vi "Target Configuration.vi"() -> ()   [LabVIEW 2019, in "LMH-LINX.lvlib"]
uses:
  <vilib>/MakerHub/LINX/LMH-LINX.lvlib
  <vilib>/MakerHub/LINX/Private/Utilties/Target Management/Install LV Data.ctl
  <vilib>/MakerHub/LINX/Private/Utilties/Target Management/Target Info.ctl
  <vilib>/MakerHub/LINX/Private/Utilties/Target Management/NIC Info.ctl
  <vilib>/MakerHub/LINX/Private/Utilties/Target Management/NIC Mode.ctl
  <vilib>/MakerHub/LINX/Private/Utilties/Install LV Events.ctl
  <vilib>/MakerHub/LINX/Private/Utilties/Target Management/Status FGV States.ctl
  <vilib>/MakerHub/LINX/Private/Utilties/Target Management/Network Settings Ctrl Refs.ctl
  <vilib>/MakerHub/LINX/Private/Utilties/Target Management/Generic FGV State.ctl
  <vilib>/Platform/browser.llb/Open URL in Default Browser (path).vi
  <vilib>/Platform/browser.llb/Open URL in Default Browser (string).vi
  <vilib>/MakerHub/Toolbox/LMH-Toolbox.lvlib
panel:
  out "Target Status 2":string
  in  "View Log":bool
  out "Status Hostname":string
  out "Target Icon":u16(ring)
  in  "Target Info":bool
  in  "Cancel All":bool=TRUE
  in  "Network Settings":bool
  in  "Installation":bool
  in  "Connection":bool=TRUE
  in  "Main OK":bool
  out "Live Status":string="Successfully connected."
  out "Error Out":errorcluster
  in  "Tab Control":T1(tab)
  out "BBB Info":bool caption="Connect your device using both USB and ethernet.\n\nUsername and password need to have sudo privileges on the target - 'debian' and 'temppwd' are the default.\n\nThe mounted USB drive includes a START.htm guide."
  out "RPI Info":bool caption="Connect your device via ethernet.\n\nUse a monitor and mouse to enable SSH.\n\nUsername and password need to have sudo privileges on the target - 'pi' and 'raspberry' are the default."
  in  "Additional installation information:":bool
  in  "Hostname or IP:":string="raspberrypi"
  in  "Username:":string="pi"
  in  "Password:":string="raspberry"
  in  "Connect":bool
  in  "Target Type":u16(ring) items=["Raspberry Pi", "BeagleBone Black"]
  out "Update Available":string="Update Available"
  in  "Install":bool
  out "Installed Version:":string
  out "Available Version:":string="14.1-9"
  in  "Example":bool
  out "EULA Link":string="here"
  in  "Network Interface:":u16(ring) items=["", "lo:", "wlan0:"]
  in  "Default gateway:":string
  in  "Subnet mask:":string
  in  "IP address:":string
  in  "Password:":string
  in  "SSID:":string
  in  "Network Settings Save":bool
  in  "Network Settings Cancel":bool
  in  "DCHP":enum32{"DHCP", "Static"}(radio)
  in  "NIC Status":string
  in  "Hostname:":string="mypi\n"
  out "Target Status":string
  out "Internet Access":string="Internet Access Confirmed"
  out "CPU Info:":string
  out "OS Version:":string="8.0\n"
  # "Wifi Settings"
  # "General Settings"
  # "IP Addresses:"
  # "Note: This utility is designed for configuring idle network adapters only.   Using it to configure an active \n           network adapter is not recommended and may result in loss of connectivity."
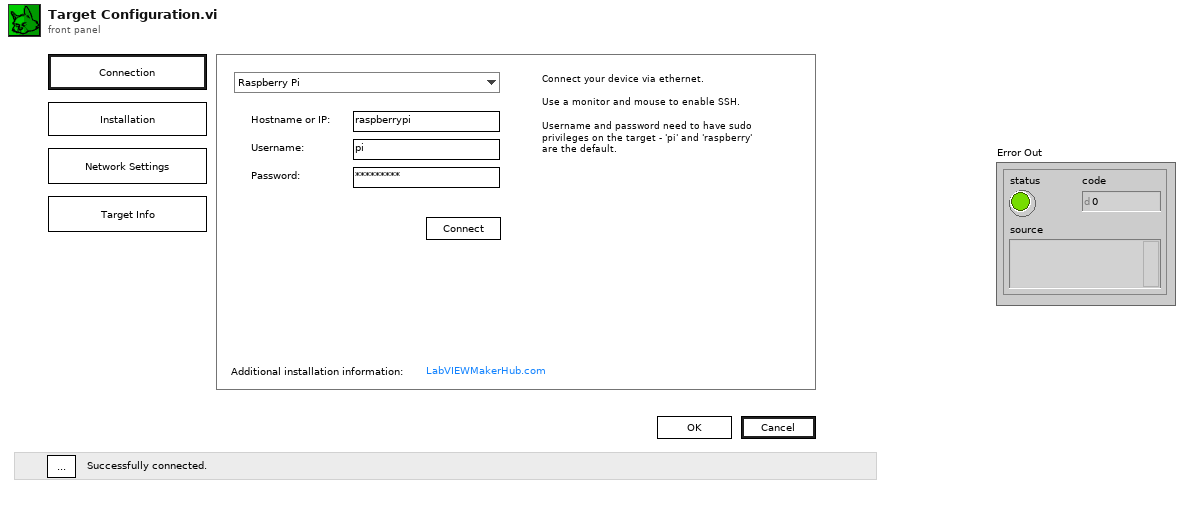
[diagram p1: front panel]
types:
  T1 = enum32{"Target", "Software", "Network", "Target Info"}
  T2 = typedef "LMH-LINX.lvlib/Install LV Events.ctl" = enum16{"Idle", "Connect", "Interrogate Device", "Pre Install", "Add MakerHub Feed", "Update Package Index", "Install LV", "Start LV", "Launch Example", "View Log", "Exit", "Update Hostname", "Menu: Target", "Menu: Install Software", "Menu: Network Settings", "Menu: Target Info", "NIC Select Change", "Menu: Network Settings Save", "Menu: Network Settings Cancel", "Menu: Cancel All"}
  T3 = typedef "LMH-LINX.lvlib/Install LV Data.ctl" = cluster{"SSH Session":refnum<k1>, "Status Log":string, "Detailed Log":string, "Credentials":cluster{"Hostname or IP":string, "Username":string, "Password":string}, "Target Info":T4, "Reboot Required?":bool}
  T4 = typedef "LMH-LINX.lvlib/Target Info.ctl" = cluster{"OS Version":string, "CPU":string, "Systemd Version":string, "Internet Access":bool, "Device Type":string, "LV Installed Ver":string, "LV Available Ver":string, "LV Upgrade Available":bool, "Hostname":string, "NIC Info":T5[]}
  T5 = typedef "LMH-LINX.lvlib/NIC Info.ctl" = cluster{"Name":string, "NIC Mode":T6, "Configured":bool, "Config IP address":string, "Config Subnet mask":string, "Config Network":string, "Config gateway":string, "Wifi":bool, "SSID":string, "Password":string, "Configuration":string, "Current IP address":string, "Current Subnet mask":string, "Current gateway":string, "Current Network":string}
  T6 = typedef "LMH-LINX.lvlib/NIC Mode.ctl" = enum16{"DHCP", "Static", "Loopback"}
  T7 = enum8{"Enabled", "Disabled", "Disabled and Grayed Out"}
  T8 = typedef "LMH-LINX.lvlib/Generic FGV State.ctl" = enum16{"Get", "Set"}
  T9 = typedef "LMH-LINX.lvlib/Network Settings Ctrl Refs.ctl" = cluster{"Hostname":refnum<vi>, "IP address":refnum<vi>, "Subnet mask":refnum<vi>, "Default Gateway":refnum<vi>, "SSID":refnum<vi>, "Password":refnum<vi>, "NIC Status":refnum<vi>, "Network Interface":refnum<vi>, "DCHP":refnum<vi>}
  T10 = typedef "LMH-LINX.lvlib/Status FGV States.ctl" = enum16{"Init", "Append", "Append History Only", "Set", "Get"}
  T11 = typedef "LMH-LINX.lvlib/Target Compatibility Warnings.ctl" = cluster{"Warning?":bool, "Details":string, "Help URL":string, "Fix It Button Name":string, "Fix It VI Ref":refnum<vi>}
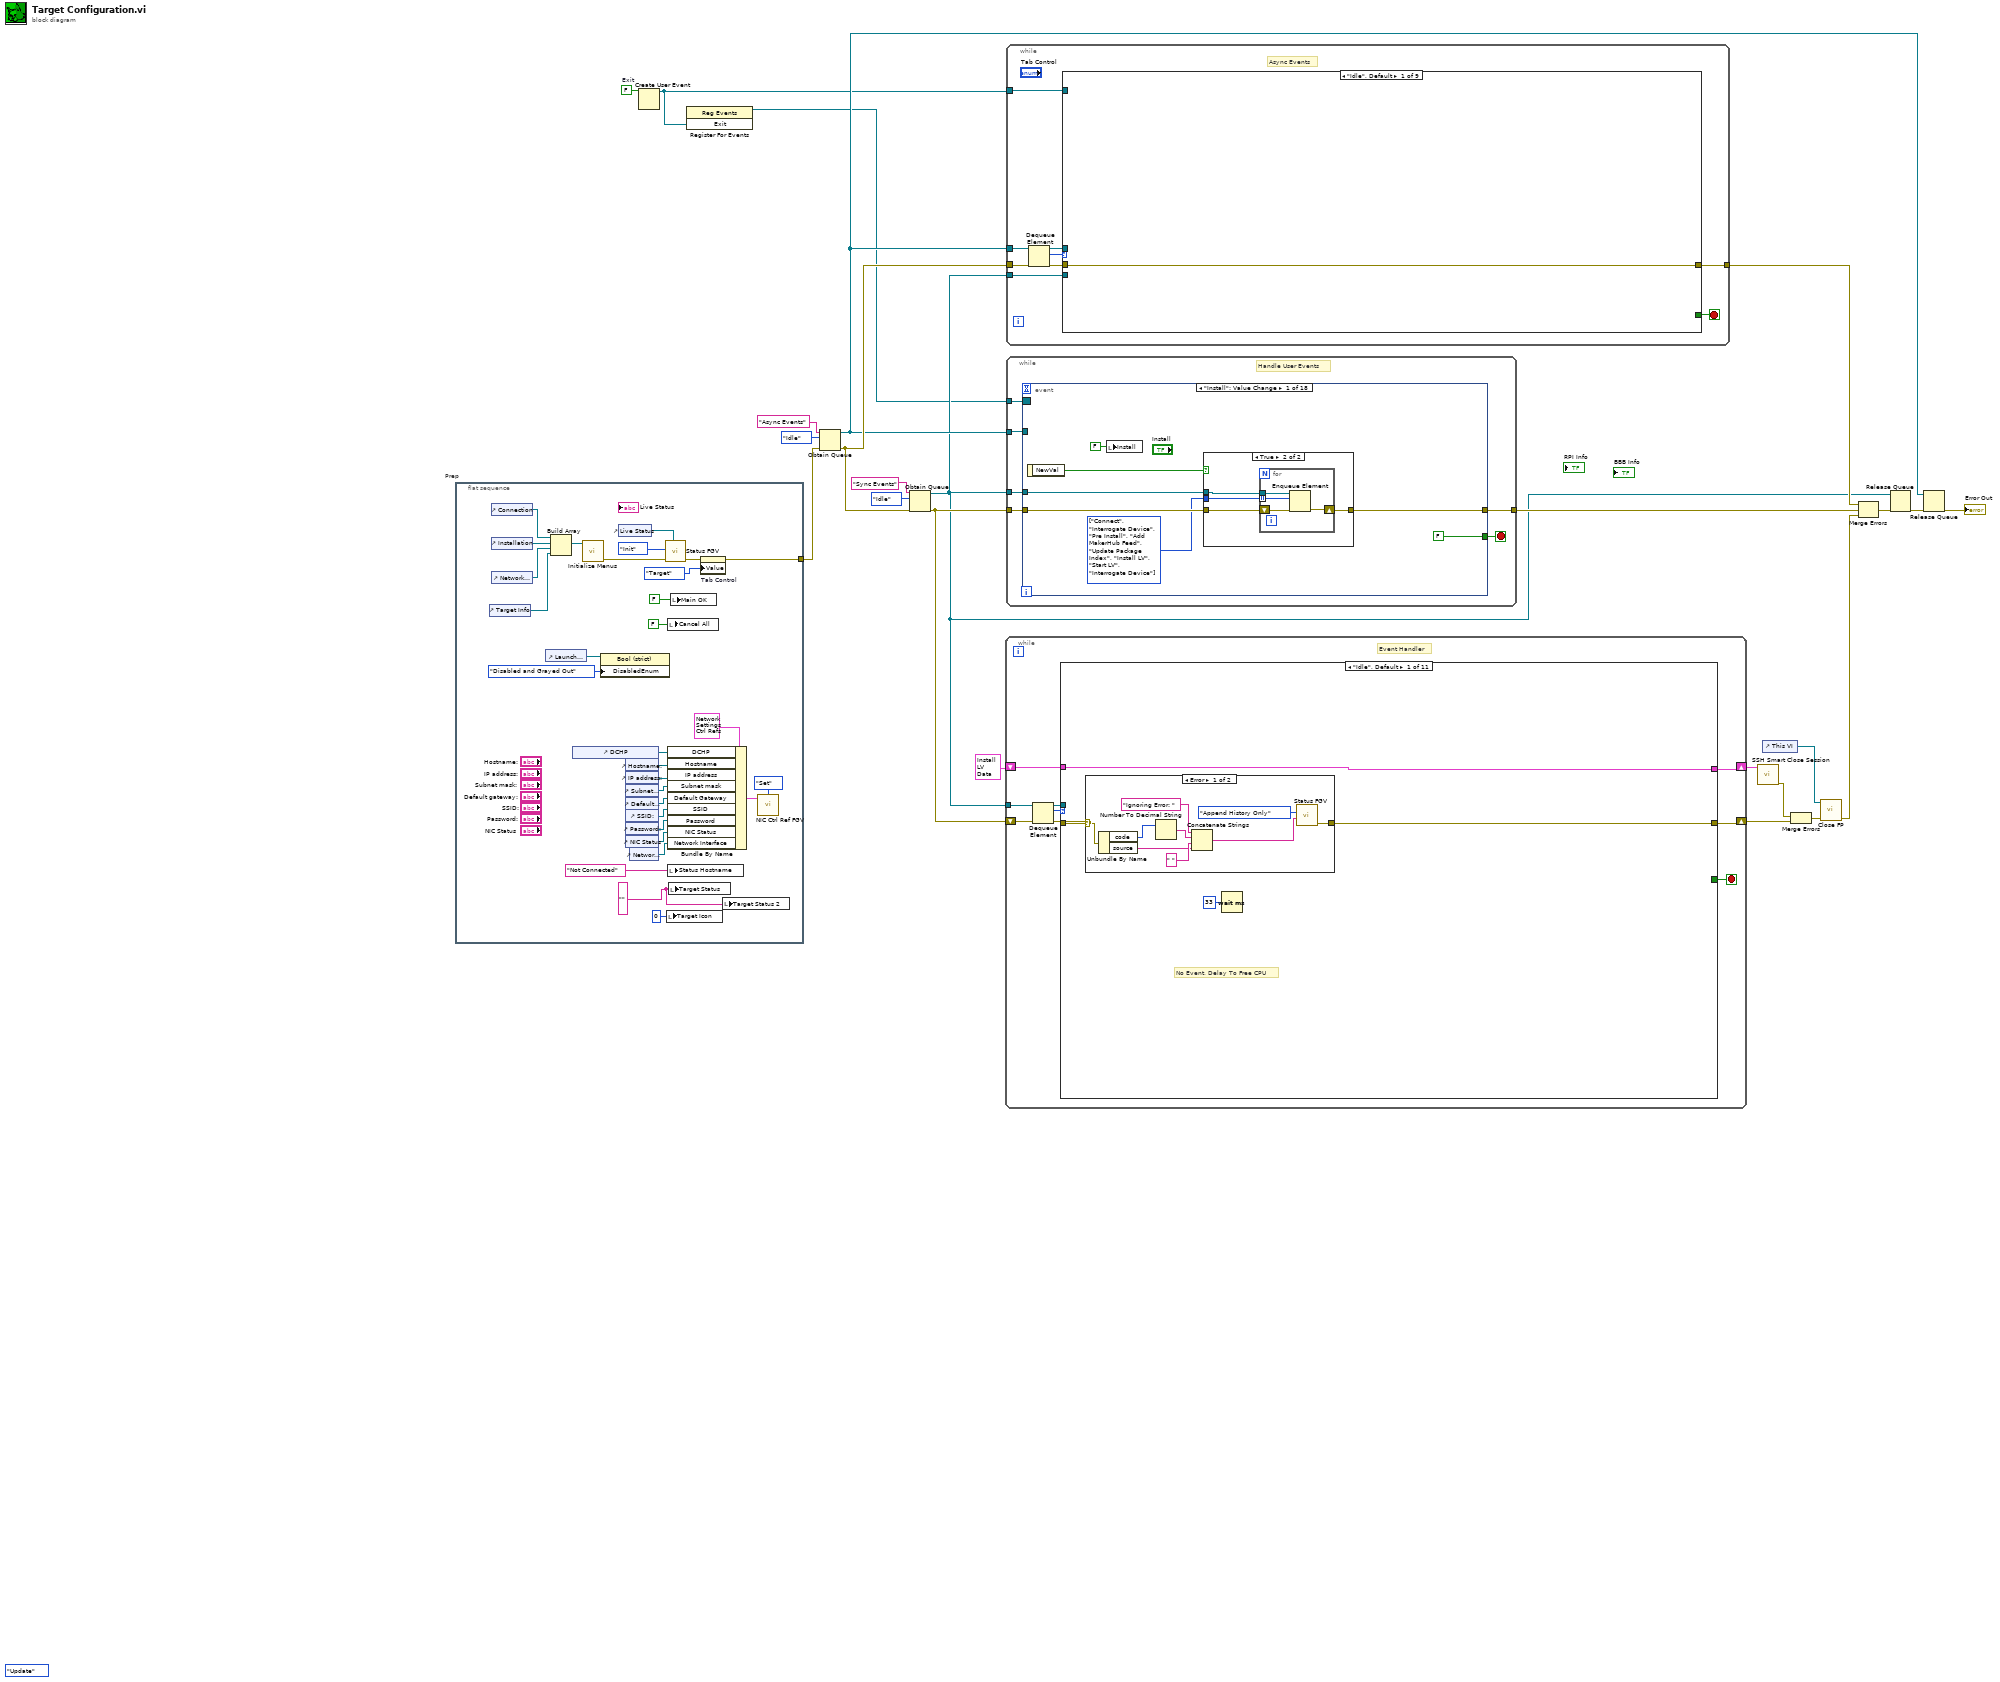
[diagram p0: block diagram]
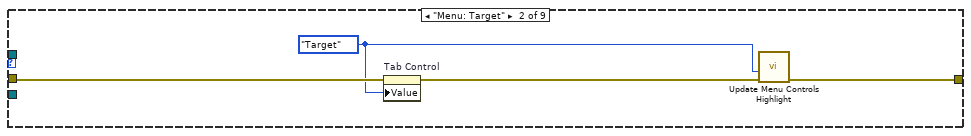
[diagram p2: hidden frame]
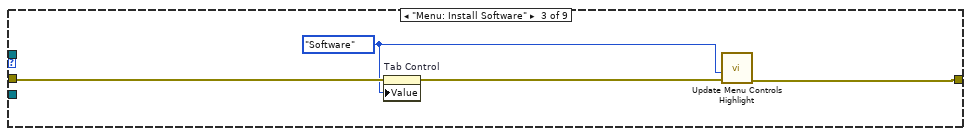
[diagram p3: hidden frame]
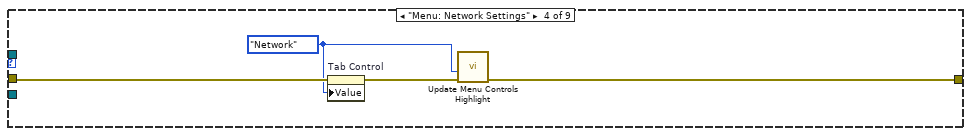
[diagram p4: hidden frame]
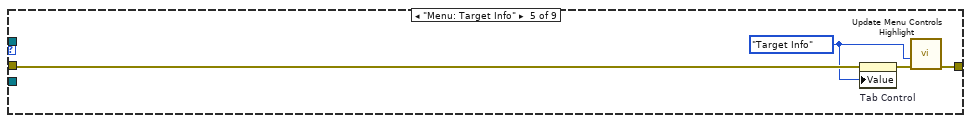
[diagram p5: hidden frame]
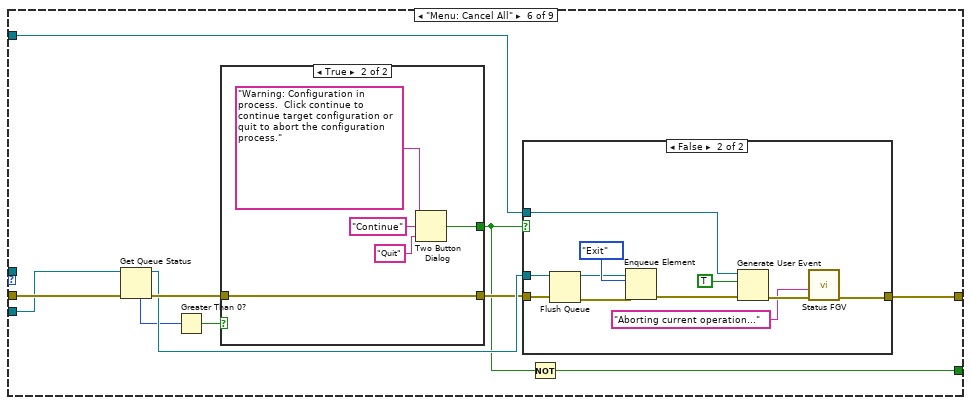
[diagram p6: hidden frame]
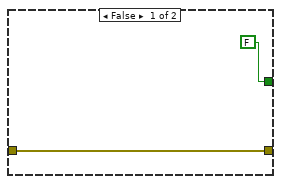
[diagram p8: hidden frame]
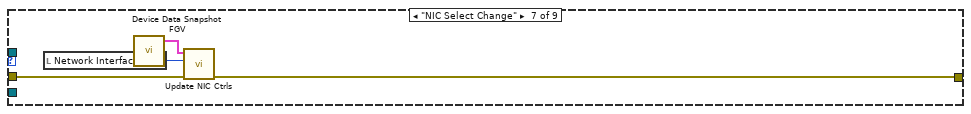
[diagram p9: hidden frame]
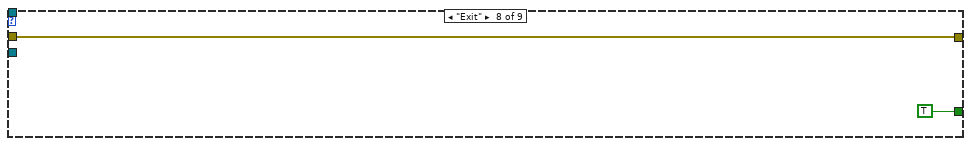
[diagram p10: hidden frame]
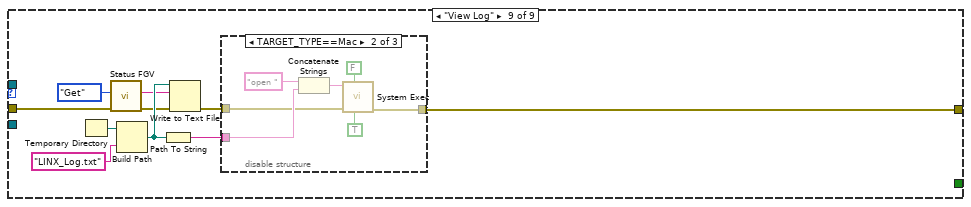
[diagram p11: hidden frame]
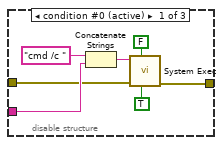
[diagram p12: hidden frame]
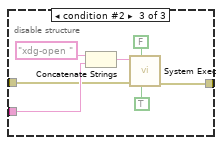
[diagram p13: hidden frame]
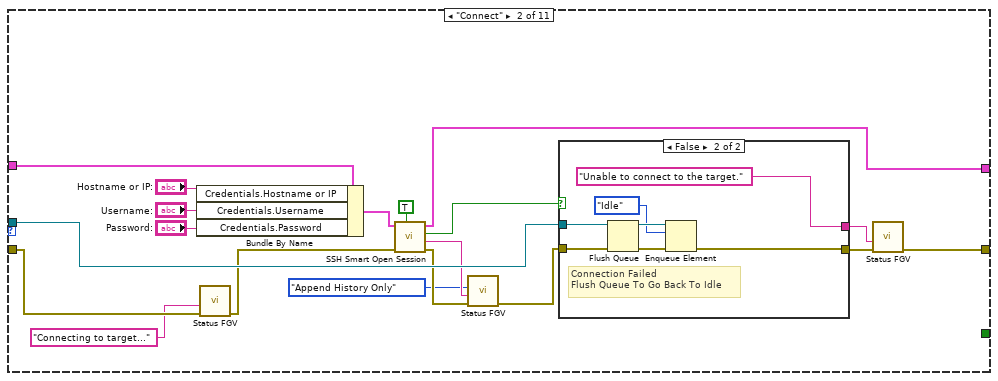
[diagram p15: hidden frame]
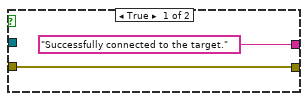
[diagram p16: hidden frame]
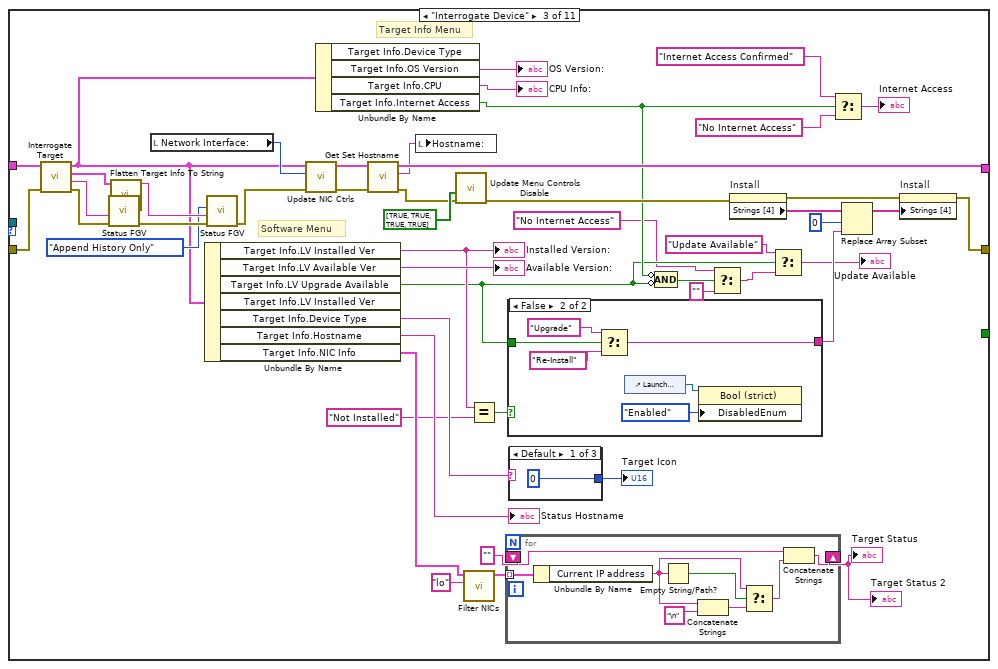
[diagram p17: hidden frame]
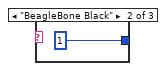
[diagram p18: hidden frame]
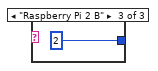
[diagram p19: hidden frame]
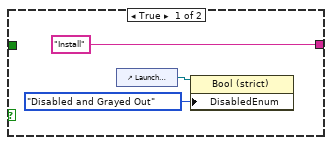
[diagram p20: hidden frame]
diagram:
  w8 = FALSE  # Exit
  (unwired) enum16{"Init", "Update"}."Update"
  n1 = flat-sequence "Prep" {
    tunnel: [w44] -> w2
    frame #0 {
      w25 = "" ("Target Stats")
      n2 = control-ref of="Target Info"() -> (w46:refnum<vi>)
      n3 = control-ref of="Connection"() -> (w51:refnum<vi>)
      n4 = control-ref of="Installation"() -> (w50:refnum<vi>)
      n5 = control-ref of="Network Settings"() -> (w49:refnum<vi>)
      n6 = control-ref of="Launch Example"() -> (w28:refnum<vi>)
      n7 = Build Array(w51, w50, w49, w46) -> (w48:refnum<vi>[])
      n8 = control-ref of="DCHP"() -> (w36:refnum<vi>)
      n9 = call <vilib>:"Initialize Menus.vi"("Menu Controls"=w48) -> ("Error Out"=w47:errorcluster)  [unwired: 10 in]
      n10 = property class="Bool (strict)"(reference=w28, "DisabledEnum"=T7."Disabled and Grayed Out" ("Disabled")) -> ()  [unwired: 1 in, 2 out]
      n11 = control-ref of="Live Status"() -> (w53:refnum<vi>)
      n12 = control-ref of="Hostname:"() -> (w31:refnum<vi>)
      n13 = control-ref of="IP address:"() -> (w37:refnum<vi>)
      n14 = control-ref of="Subnet mask:"() -> (w38:refnum<vi>)
      n15 = control-ref of="Default gateway:"() -> (w39:refnum<vi>)
      n16 = control-ref of="SSID:"() -> (w40:refnum<vi>)
      n17 = control-ref of="Password:"() -> (w41:refnum<vi>)
      n18 = control-ref of="NIC Status"() -> (w42:refnum<vi>)
      n19 = control-ref of="Network Interface:"() -> (w34:refnum<vi>)
      n20 = call <vilib>:"Status FGV.vi"("Live Status Ref"=w53, "Error In"=w47, "Status FGV State"=Status_FGV_States."Init") -> ("Error Out"=w45:errorcluster)  [unwired: 6 in, 2 out]
      n21 = local write "Target Icon"(u16 0 ("Target Icon")) -> ()
      n22 = local write "Cancel All"(FALSE ("Stop Button")) -> ()
      n23 = Bundle By Name(cluster=T9 {"Hostname"=refnum, "IP address"=refnum, "Subnet mask"=refnum, "Default Gateway"=refnum, "SSID"=refnum, "Password"=refnum, "NIC Status"=refnum, "Network Interface"=refnum, "DCHP"=refnum} ("Network Settings Ctrl Refs"), "DCHP"=w36, "Hostname"=w31, "IP address"=w37, "Subnet mask"=w38, "Default Gateway"=w39, "SSID"=w40, "Password"=w41, "NIC Status"=w42, "Network Interface"=w34) -> (w33:T9)
      n24 = local write "Status Hostname"("Not Connected") -> ()
      n25 = local write "Target Status"(w25) -> ()
      n26 = local write "Main OK"(FALSE ("Stop Button")) -> ()
      n27 = property on="Tab Control" class="TabCtl (strict)"(error in=w45, "Value"=T1."Target" ("Tab Control")) -> (error out=w44:errorcluster)  [unwired: 1 in, 1 out]
      n28 = local write "Target Status 2"(w25) -> ()
      n29 = call <vilib>:"NIC Ctrl Ref FGV.vi"("Network Settings Ctrl Refs"=w33, "FGV State"=Generic_FGV_State."Set") -> ()  [unwired: 2 in, 1 out]
    }
  }
  n30 = Create User Event(user event datatype=w8) -> (user event=w6:refnum<user-event>)  [unwired: 1 in, 1 out]
  n31 = register-events(w6) -> (reference out=w7:refnum<event-registration>)  [unwired: 2 in, 1 out]
  n32 = Obtain Queue(name (unnamed)="Async Events", element data type=Install_LV_Events."Idle" ("Install LV Support State"), error in (no error)=w2) -> (queue out=w10:refnum<queue>, error out=w14:errorcluster)  [unwired: 2 in, 1 out]
  n33 = Obtain Queue(name (unnamed)="Sync Events", element data type=Install_LV_Events."Idle" ("Install LV Support State"), error in (no error)=w14) -> (queue out=w9:refnum<queue>, error out=w23:errorcluster)  [unwired: 2 in, 1 out]
  n34 = while {
    shift-right: [w62] -> w3
    shift-left: w23 -> [w60]
    tunnel: w9 -> [w61]
    shift-right: [w57] -> w17
    shift-left: T3 {"SSH Session"=refnum, "Status Log"="", "Detailed Log"="", "Credentials"={"Hostname or IP"="", "Username"="", "Password"=""}, "Target Info"={"OS Version"="", "CPU"="", "Systemd Version"="", "Internet Access"=FALSE, "Device Type"="", "LV Installed Ver"="", "LV Available Ver"="", "LV Upgrade Available"=FALSE, "Hostname"="", "NIC Info"=[]}, "Reboot Required?"=FALSE} ("Install LV Data") -> [w56]
    stop <- w63 stop-if-true
    # "Event Handler"
    n35 = Dequeue Element(queue=w61, error in (no error)=w60) -> (queue out=w55:refnum<queue>, element=w58:T2, error out=w59:errorcluster)  [unwired: 1 in, 1 out]
    n36 = case shown="\"Idle\", Default" w58 {
      tunnel: [w64 w79 w118 w179 w215 w231 w243 w252 w266 w304 w330] -> w62
      tunnel: w59 -> [w65 w83 w154 w183 w227 w237 w246 w255 w264 w305 w330]
      tunnel: [_ _ _ _ _ _ _ _ _ _ TRUE] -> w63
      tunnel: [w66 w85 w134 w178 w222 w229 w238 w247 w260 w298 w329] -> w57
      tunnel: w56 -> [w66 w87 w147 w177 w223 w230 w239 w248 w262 w299 w329]
      tunnel: w55 -> [_ w94 _ w184 w217 _ _ _ _ w300 _]
      frame "Idle", Default {
        # "No Event, Delay To Free CPU"
        n37 = case shown="Error" w65 {
          selector: w65 -> [w75 w77]
          tunnel: [w76 w77] -> w64
          frame Error {
            n38 = Unbundle By Name(w75) -> ("code"=w73:i32, "source"=w70:string)
            n39 = Number To Decimal String(number=w73) -> (decimal integer string=w72:string)  [unwired: 1 in]
            n40 = Concatenate Strings("Ignoring Error: " ("Status"), w72, " " ("string"), w70) -> (w69:string)
            n41 = call <vilib>:"Status FGV.vi"("Status"=w69, "Status FGV State"=Status_FGV_States."Append History Only") -> ("Error Out"=w76:errorcluster)  [unwired: 7 in, 2 out]
          }
          frame No Error {
          }
        }
        n42 = Wait (ms)(milliseconds to wait=u32 33) -> ()  [unwired: 1 out]
      }
      frame "Connect" {
        n43 = Bundle By Name(cluster=w87, "Credentials.Hostname or IP"="Hostname or IP:", "Credentials.Username"="Username:", "Credentials.Password"="Password:") -> (w86:T3)
        n44 = call <vilib>:"Status FGV.vi"("Error In"=w83, "Status"="Connecting to target...") -> ("Error Out"=w82:errorcluster)  [unwired: 7 in, 2 out]
        n45 = call <vilib>:"SSH Smart Open Session.vi"("Force Reconnect?"=TRUE, "Error In"=w82, "Install LV Data in"=w86) -> ("Error Out"=w93:errorcluster, "Status"=w91:string, "Connected?"=w95:bool, "Install LV Data out"=w85:T3)  [unwired: 5 in]
        n46 = call <vilib>:"Status FGV.vi"("Error In"=w93, "Status"=w91, "Status FGV State"=Status_FGV_States."Append History Only") -> ("Error Out"=w92:errorcluster)  [unwired: 6 in, 2 out]
        n47 = case shown="False" w95 {
          tunnel: w94 -> [_ w105]
          tunnel: w92 -> [w98 w101]
          tunnel: [w98 w100] -> w80
          tunnel: ["Successfully connected to the target." ("Status") "Unable to connect to the target." ("Status")] -> w78
          frame True {
          }
          frame False {
            # "Connection Failed\nFlush Queue To Go Back To Idle"
            n48 = Flush Queue(queue=w105, error in (no error)=w101) -> (queue out=w103:refnum<queue>, error out=w104:errorcluster)  [unwired: 1 out]
            n49 = Enqueue Element(queue=w103, element=Install_LV_Events."Idle", error in (no error)=w104) -> (error out=w100:errorcluster)  [unwired: 1 in, 2 out]
          }
        }
        n50 = call <vilib>:"Status FGV.vi"("Error In"=w80, "Status"=w78) -> ("Error Out"=w79:errorcluster)  [unwired: 7 in, 2 out]
      }
      frame "Interrogate Device" {
        # "Software Menu"
        # "Target Info Menu"
        n51 = call <vilib>:"Interrogate Target.vi"("Error In"=w154, "Install LV Data"=w147) -> ("Error Out"=w153:errorcluster, "Status"=w152:string, "Target Info"=w151:T4, "Install LV Data"=w137:T3)  [unwired: 6 in]
        n52 = call <vilib>:"Status FGV.vi"("Error In"=w153, "Status"=w152) -> ("Error Out"=w149:errorcluster)  [unwired: 7 in, 2 out]
        n53 = call <vilib>:"Flatten Target Info To String.vi"("Target Info"=w151) -> ("Target Info String"=w150:string)  [unwired: 10 in]
        n54 = local read "Network Interface:"() -> (w139:u16)
        n55 = Unbundle By Name(w137) -> ("Target Info.LV Installed Ver"=w122:string, "Target Info.LV Available Ver"=→"Available Version:":string, "Target Info.LV Upgrade Available"=w111:bool, "Target Info.Device Type"=w130:string, "Target Info.Hostname"=→"Status Hostname":string, "Target Info.NIC Info"=w127:T5[])  [unwired: 1 out]
        "Installed Version:" <- w122
        n56 = call <vilib>:"Status FGV.vi"("Error In"=w149, "Status"=w150, "Status FGV State"=Status_FGV_States."Append History Only") -> ("Error Out"=w138:errorcluster)  [unwired: 6 in, 2 out]
        n57 = call <vilib>:"Update NIC Ctrls.vi"("Error In"=w138, "Selected NIC"=w139, "Install LV Data"=w137) -> ("Error Out"=w135:errorcluster, "Install LV Data"=w136:T3)  [unwired: 7 in]
        n58 = Unbundle By Name(w137) -> ("Target Info.OS Version"=→"OS Version:":string, "Target Info.CPU"=→"CPU Info:":string, "Target Info.Internet Access"=w112:bool)  [unwired: 1 out]
        n59 = call <vilib>:"Get Set Hostname.vi"("Error In"=w135, "Install LV Data"=w136) -> ("Error Out"=w131:errorcluster, "Hostname"=w133:string, "Install LV Data"=w134:T3)  [unwired: 7 in]
        n60 = local write "Hostname:"(w133) -> ()
        n61 = call <vilib>:"Update Menu Controls Disable.vi"("Error In"=w131, "Enabled?"=bool[] [TRUE, TRUE, TRUE, TRUE]) -> ("Error Out"=w119:errorcluster)  [unwired: 9 in]
        n62 = call <vilib>:"Filter NICs.vi"("NIC Name"="lo", "NIC Configs"=w127) -> ("NIC Configs"=w126:T5[])  [unwired: 8 in, 1 out]
        n63 = Equal?(x=w122, y="Not Installed") -> (x = y?=w121:bool)
        n64 = for {
          tunnel: w126 -> [w162] mode=indexing
          shift-right: [w155] -> w106
          shift-left: "" -> [w161]
          n65 = Unbundle By Name(w162) -> ("Current IP address"=w159:string)
          n66 = Empty String/Path?(string/path=w159) -> (empty?=w160:bool)
          n67 = Concatenate Strings(w159, "\n") -> (w157:string)
          n68 = Select(t=w159, s=w160, f=w157) -> (s? t:f=w156:string)
          n69 = Concatenate Strings(w161, w156) -> (w155:string)
        }
        "Target Status" <- w106
        "Target Status 2" <- w106
        n70 = case shown="False" w121 {
          tunnel: ["Install" w171] -> w141
          tunnel: w111 -> [_ w174]
          frame True {
            n71 = control-ref of="Launch Example"() -> (w166:refnum<vi>)
            n72 = property class="Bool (strict)"(reference=w166, "DisabledEnum"=T7."Disabled and Grayed Out" ("Disabled")) -> ()  [unwired: 1 in, 2 out]
          }
          frame False {
            n73 = Select(t="Upgrade", s=w174, f="Re-Install") -> (s? t:f=w171:string)
            n74 = control-ref of="Launch Example"() -> (w169:refnum<vi>)
            n75 = property class="Bool (strict)"(reference=w169, "DisabledEnum"=T7."Enabled" ("Disabled")) -> ()  [unwired: 1 in, 2 out]
          }
        }
        n76 = case shown="Default" w130 {
          tunnel: [u16 0 ("Target Icon") u16 1 ("Target Icon") u16 2 ("Target Icon")] -> w128
          frame Default {
          }
          frame "BeagleBone Black" {
          }
          frame "Raspberry Pi 2 B" {
          }
        }
        "Target Icon" <- w128
        n77 = Compound Arithmetic op=AND(invert w112, invert w111) -> (w107:bool)
        n78 = Select(t="No Internet Access" ("Internet Access"), s=w107, f="") -> (s? t:f=w110:string)
        n79 = property on="Install" class="Bool (strict)"(error in=w119) -> (error out=w120:errorcluster, "Strings [4]"=w143:string[])  [unwired: 1 in, 1 out]
        n80 = Select(t="Update Available" ("Update Available"), s=w111, f=w110) -> (s? t:f=→"Update Available":string)
        n81 = Select(t="Internet Access Confirmed" ("Internet Access"), s=w112, f="No Internet Access" ("Internet Access")) -> (s? t:f=→"Internet Access":string)
        n82 = Replace Array Subset(array=w143, new element=w141, index=0) -> (w142:string[])
        n83 = property on="Install" class="Bool (strict)"(error in=w120, "Strings [4]"=w142) -> (error out=w118:errorcluster)  [unwired: 1 in, 1 out]
      }
      frame "Pre Install" {
        # "Do any device specific pre-install prep here."
        n84 = call <vilib>:"Generate Target Compatibility Report.vi"("Error In"=w183, "Install LV Data"=w177) -> ("Error Out"=w180:errorcluster, "Can Continue?"=w181:bool, "Warnings"=w182:T11[], "Install LV Data"=w176:T3)  [unwired: 6 in]
        n85 = Array Size(array=w182) -> (size(s)=w188:i32)
        n86 = Greater Than 0?(x=w188) -> (x > 0?=w187:bool)
        n87 = case shown="True" w187 {
          tunnel: [w204 w211] -> w186
          tunnel: [TRUE ("Continue?") w210] -> w185
          tunnel: w180 -> [w204 w209]
          tunnel: w182 -> [_ w208]
          tunnel: w181 -> [_ w207]
          tunnel: w176 -> [w202 w206]
          tunnel: [w202 w205] -> w175
          frame False {
          }
          frame True {
            n88 = call <vilib>:"Show Compatibility Warnings.vi"("Error In"=w209, "Can Continue?"=w207, "Warnings"=w208, "Install LV Data"=w206) -> ("Error Out"=w211:errorcluster, "Continue?"=w210:bool, "Install LV Data"=w205:T3)  [unwired: 4 in, 1 out]
          }
        }
        n89 = case shown="True" w185 {
          tunnel: w186 -> [w192 w198]
          tunnel: [w191 w194] -> w179
          tunnel: w184 -> [_ w196]
          tunnel: [w190 w193] -> w178
          tunnel: w175 -> [w189 w193]
          frame True {
            n90 = call <vilib>:"Device Pre Install Tasks.vi"("Error In"=w192, "Install LV Data"=w189) -> ("Error Out"=w191:errorcluster, "Install LV Data"=w190:T3)  [unwired: 8 in]
          }
          frame False {
            # "Do No Install Software\nFlush Queue To Go Back To Idle"
            n91 = call <vilib>:"Status FGV.vi"("Error In"=w198, "Status"="Install cancelled.") -> ("Error Out"=w195:errorcluster)  [unwired: 7 in, 2 out]
            n92 = Flush Queue(queue=w196, error in (no error)=w195) -> (queue out=w200:refnum<queue>, error out=w201:errorcluster)  [unwired: 1 out]
            n93 = Enqueue Element(queue=w200, element=Install_LV_Events."Idle", error in (no error)=w201) -> (error out=w194:errorcluster)  [unwired: 1 in, 2 out]
          }
        }
      }
      frame "Menu: Network Settings Save" {
        n94 = local read "Network Interface:"() -> (w226:u16)
        n95 = local read "Hostname:"() -> (w219:string)
        n96 = call <vilib>:"Status FGV.vi"("Error In"=w227, "Status"="Saving Network Configuration...") -> ("Error Out"=w221:errorcluster)  [unwired: 7 in, 2 out]
        n97 = call <vilib>:"Get Set Hostname.vi"("Error In"=w221, "Set"=TRUE, "Hostname"=w219, "Install LV Data"=w223) -> ("Error Out"=w225:errorcluster, "Hostname"=w218:string, "Install LV Data"=w224:T3)  [unwired: 5 in]
        n98 = local write "Hostname:"(w218) -> ()
        n99 = call <vilib>:"Save NIC Settings.vi"("Network Interface:"=w226, "Error In"=w225, "Install LV Data"=w224) -> ("Error Out"=w214:errorcluster, "Install LV Data"=w222:T3)  [unwired: 7 in]
        n100 = call <vilib>:"Status FGV.vi"("Error In"=w214, "Status"="Network settings saved.  Target may need to be rebooted before new settings are applied.") -> ("Error Out"=w213:errorcluster)  [unwired: 7 in, 2 out]
        n101 = Enqueue Element(queue=w217, element=Install_LV_Events."Interrogate Device", error in (no error)=w213) -> (error out=w215:errorcluster)  [unwired: 1 in, 2 out]
      }
      frame "Add MakerHub Feed" {
        n102 = call <vilib>:"Status FGV.vi"("Error In"=w237, "Status"="Adding MakerHub feed...") -> ("Error Out"=w236:errorcluster)  [unwired: 7 in, 2 out]
        n103 = call <vilib>:"Add MakerHub Feed.vi"("Error In"=w236, "Install LV Data"=w230) -> ("Error Out"=w234:errorcluster, "Log"=w233:string, "Install LV Data"=w229:T3)  [unwired: 7 in]
        n104 = call <vilib>:"Status FGV.vi"("Error In"=w234, "Status"=w233, "Status FGV State"=Status_FGV_States."Append History Only") -> ("Error Out"=w231:errorcluster)  [unwired: 6 in, 2 out]
      }
      frame "Update Package Index" {
        n105 = call <vilib>:"Status FGV.vi"("Error In"=w246, "Status"="Updating package index.  This may take over 30 seconds depending on your internet speed...") -> ("Error Out"=w242:errorcluster)  [unwired: 7 in, 2 out]
        n106 = call <vilib>:"Update Package List.vi"("Error In"=w242, "Install LV Data"=w239) -> ("Error Out"=w241:errorcluster, "Log"=w240:string, "Install LV Data"=w238:T3)  [unwired: 7 in]
        n107 = call <vilib>:"Status FGV.vi"("Error In"=w241, "Status"=w240, "Status FGV State"=Status_FGV_States."Append History Only") -> ("Error Out"=w243:errorcluster)  [unwired: 6 in, 2 out]
      }
      frame "Install LV" {
        n108 = call <vilib>:"Status FGV.vi"("Error In"=w255, "Status"="Installing LabVIEW...") -> ("Error Out"=w249:errorcluster)  [unwired: 7 in, 2 out]
        n109 = call <vilib>:"Install LV Support.vi"("Error In"=w249, "Install LV Data"=w248) -> ("Error Out"=w251:errorcluster, "Log"=w250:string, "Install LV Data"=w247:T3)  [unwired: 7 in]
        n110 = call <vilib>:"Status FGV.vi"("Error In"=w251, "Status"=w250, "Status FGV State"=Status_FGV_States."Append History Only") -> ("Error Out"=w252:errorcluster)  [unwired: 6 in, 2 out]
      }
      frame "Start LV" {
        n111 = Unbundle By Name(w262) -> ("Reboot Required?"=w265:bool)
        n112 = case shown="True" w265 {
          tunnel: w264 -> [w291 w297]
          tunnel: [w291 w296] -> w263
          tunnel: w262 -> [w292 w295]
          tunnel: [w292 w294] -> w261
          tunnel: [TRUE ("Connected?") w293] -> w259
          frame False {
          }
          frame True {
            n113 = call <vilib>:"Reboot Target.vi"("Error In"=w297, "Install LV Data"=w295) -> ("Error Out"=w296:errorcluster, "Connected?"=w293:bool, "Install LV Data"=w294:T3)  [unwired: 7 in]
          }
        }
        n114 = case shown="True" w259 {
          tunnel: [w268 w277] -> w266
          tunnel: w263 -> [w268 w276]
          tunnel: w261 -> [w267 w275]
          tunnel: [w267 w274] -> w260
          tunnel: Status_FGV_States."Append History Only" ("Status FGV State") -> [_ w271]
          tunnel: "Checking target status..." ("Status") -> [_ w270]
          tunnel: "Installation completed successfully.  Click Launch Example to get started." ("Status") -> [_ w269]
          frame False {
            # "Unable to reconnect to target..."
          }
          frame True {
            n115 = call <vilib>:"Status FGV.vi"("Error In"=w276, "Status"=w270) -> ("Error Out"=w280:errorcluster)  [unwired: 7 in, 2 out]
            n116 = call <vilib>:"Start LabVIEW.vi"("Error In"=w280, "Install LV Data"=w275) -> ("Error Out"=w279:errorcluster, "Log"=w278:string, "LV Running?"=w272:bool, "Install LV Data"=w274:T3)  [unwired: 6 in]
            n117 = call <vilib>:"Status FGV.vi"("Error In"=w279, "Status"=w278, "Status FGV State"=w271) -> ("Error Out"=w273:errorcluster)  [unwired: 6 in, 2 out]
            n118 = case shown="True" w272 {
              tunnel: [w283 w289] -> w277
              tunnel: w273 -> [w281 w286]
              tunnel: w269 -> [_ w284]
              frame False {
                n119 = call <vilib>:"Status FGV.vi"("Error In"=w281, "Status"="Installation failed.  If this is the first time the installation has failed try again.  If this error persists search, then post on the LabVIEW MakerHub forumsat labviewmakerhub.com/forums/linx.") -> ("Error Out"=w283:errorcluster)  [unwired: 7 in, 2 out]
              }
              frame True {
                n120 = control-ref of="Launch Example"() -> (w288:refnum<vi>)
                n121 = property class="Bool (strict)"(reference=w288, error in=w286, "DisabledEnum"=T7."Enabled" ("Disabled")) -> (error out=w285:errorcluster)  [unwired: 1 out]
                n122 = call <vilib>:"Status FGV.vi"("Error In"=w285, "Status"=w284) -> ("Error Out"=w289:errorcluster)  [unwired: 7 in, 2 out]
              }
            }
          }
        }
      }
      frame "Launch Example" {
        n123 = Unbundle By Name(w299) -> ("Target Info.Device Type"=w303:string)
        n124 = Equal?(x=w303, y="") -> (x = y?=w302:bool)
        n125 = case shown="False" w302 {
          tunnel: w305 -> [w312 w323]
          tunnel: [w307 w321] -> w304
          tunnel: w299 -> [w306 w318]
          tunnel: w300 -> [w311 _]
          tunnel: [w306 w318] -> w298
          frame True {
            w308 = T2[] [enum."Connect", enum."Interrogate Device", enum."Launch Example", enum."Exit"] items=["Idle", "Connect", "Interrogate Device", "Pre Install", "Add MakerHub Feed", "Update Package Index", "Install LV", "Start LV", "Launch Example", "View Log", "Exit", "Update Hostname", "Menu: Target", "Menu: Install Software", "Menu: Network Settings", "Menu: Target Info", "NIC Select Change", "Menu: Network Settings Save", "Menu: Network Settings Cancel", "Menu: Cancel All"] ("remaining elements")
            n126 = Flush Queue(queue=w311, error in (no error)=w312) -> (queue out=w309:refnum<queue>, error out=w310:errorcluster)  [unwired: 1 out]
            n127 = for {
              shift-right: [w316] -> w307
              shift-left: w310 -> [w317]
              shift-right: [w315] -> _
              shift-left: w309 -> [w314]
              tunnel: w308 -> [w313] mode=indexing
              n128 = Enqueue Element(queue=w314, element=w313, error in (no error)=w317) -> (queue out=w315:refnum<queue>, error out=w316:errorcluster)  [unwired: 1 in, 1 out]
            }
          }
          frame False {
            n129 = control-ref of="This VI"() -> (w324:refnum<vi>)
            n130 = property class="VI"(reference=w324, error in=w323, "FP:RunTransparently"=TRUE ("Front Panel Window:Run VI Transparently"), "FP:Transparency"=u8 100 ("Front Panel Window:Transparency")) -> (error out=w322:errorcluster)  [unwired: 1 out]
            n131 = Unbundle By Name(w318) -> ("Target Info.Device Type"=w326:string, "Credentials.Hostname or IP"=w325:string)
            n132 = call <vilib>:"Status FGV.vi"("Error In"=w322, "Status"="Creating example project.") -> ("Error Out"=w327:errorcluster)  [unwired: 7 in, 2 out]
            n133 = call <vilib>:"Script Example Project.vi"("Error In"=w327, "Hostname or IP"=w325, "Device Name"=w326) -> ("Error Out"=w321:errorcluster)  [unwired: 8 in]
          }
        }
      }
      frame "Exit" {
      }
    }
  }
  n134 = while {
    tunnel: w10 -> [w334]
    tunnel: w9 -> [w333]
    tunnel: w23 -> [w337]
    tunnel: [w336] -> w18
    tunnel: w7 -> [w332]
    stop <- w335 stop-if-true
    # "Handle User Events"
    n135 = event shown="[0] \"Install\": Value Change" {
      selector: w332 -> [_ _ _ _ _ _ _ _ _ _ _ _ _ _ _ _ _ _]
      dyn-events: _ -> [_ _ _ _ _ _ _ _ _ _ _ _ _ _ _ _ _ _]
      timeout: _ -> [_ _ _ _ _ _ _ _ _ _ _ _ _ _ _ _ _ _]
      tunnel: [w341 w356 w373 w376 w381 w395 w404 w408 w412 w420 w422 w425 w431 w437 w443 w459 w471 w473] -> w336
      tunnel: w337 -> [w342 w358 w372 w377 w389 w394 w405 w409 w413 w416 w421 w428 w435 w440 w444 w459 w470 w473]
      tunnel: [FALSE TRUE FALSE FALSE TRUE FALSE _ _ _ _ _ _ _ _ _ _ _ TRUE] -> w335
      tunnel: w334 -> [_ w359 _ w374 w382 _ w402 w406 w410 w418 w424 _ _ w439 _ _ _ _]
      tunnel: w333 -> [w338 w354 _ _ w384 w392 _ _ _ w414 _ w427 w434 _ _ _ _ _]
      event "Install": Value Change {
        w339 = T2[] [enum."Connect", enum."Interrogate Device", enum."Pre Install", enum."Add MakerHub Feed", enum."Update Package Index", enum."Install LV", enum."Start LV", enum."Interrogate Device"] items=["Idle", "Connect", "Interrogate Device", "Pre Install", "Add MakerHub Feed", "Update Package Index", "Install LV", "Start LV", "Launch Example", "View Log", "Exit", "Update Hostname", "Menu: Target", "Menu: Install Software", "Menu: Network Settings", "Menu: Target Info", "NIC Select Change", "Menu: Network Settings Save", "Menu: Network Settings Cancel", "Menu: Cancel All"]
        n136 = event-data() -> ("NewVal"=w340:bool)  [unwired: 1 in]
        n137 = local write "Install"(FALSE ("Install")) -> ()
        n138 = case shown="True" w340 {
          tunnel: w342 -> [w345 w349]
          tunnel: [w345 w348] -> w341
          tunnel: w339 -> [_ w347]
          tunnel: w338 -> [_ w346]
          frame False {
            # "Ignore Change \nto False"
          }
          frame True {
            n139 = for {
              shift-right: [w352] -> w348
              shift-left: w349 -> [w353]
              tunnel: w347 -> [w351] mode=indexing
              tunnel: w346 -> [w350]
              n140 = Enqueue Element(queue=w350, element=w351, error in (no error)=w353) -> (error out=w352:errorcluster)  [unwired: 1 in, 2 out]
            }
          }
        }
      }
      event "Main OK": Value Change {
        w355 = Install_LV_Events."Exit" ("element")
        n141 = event-data() -> ()  [unwired: 1 in, 1 out]
        n142 = local write "Main OK"(FALSE ("Stop Button")) -> ()
        n143 = Enqueue Element(queue=w354, element=w355, error in (no error)=w358) -> (error out=w357:errorcluster)  [unwired: 1 in, 2 out]
        n144 = Enqueue Element(queue=w359, element=w355, error in (no error)=w357) -> (error out=w356:errorcluster)  [unwired: 1 in, 2 out]
      }
      event "EULA Link": Mouse Up {
        n145 = event-data() -> ()  [unwired: 1 in, 1 out]
        n146 = call <vilib>:"Get Current LV Dir.vi"() -> ("This LV Directory"=w363:path)  [unwired: 10 in, 1 out]
        n147 = Build Path(base path=w363, name or relative path="resource") -> (appended path=w370:path)
        n148 = Build Path(base path=w370, name or relative path="Framework") -> (appended path=w369:path)
        n149 = Build Path(base path=w369, name or relative path="Providers") -> (appended path=w368:path)
        n150 = Build Path(base path=w368, name or relative path="LINX Provider EULA.txt") -> (appended path=w362:path)
        n151 = call-poly <vilib>:"Open URL in Default Browser.vi"("error in (no error)"=w372, "path"=w362) -> ("error out"=w373:errorcluster)  [unwired: 4 in, 1 out]
      }
      event "View Log": Value Change {
        n152 = event-data() -> ()  [unwired: 1 in, 1 out]
        n153 = local write "View Log"(FALSE ("View Log")) -> ()
        n154 = Enqueue Element(queue=w374, element=Install_LV_Events."View Log", error in (no error)=w377) -> (error out=w376:errorcluster)  [unwired: 1 in, 2 out]
      }
      event "Example": Value Change {
        n155 = event-data() -> ()  [unwired: 1 in, 1 out]
        n156 = local write "Example"(FALSE ("Launch Example")) -> ()
        n157 = Enqueue Element(queue=w384, element=Install_LV_Events."Launch Example" ("Install LV Support State"), error in (no error)=w389) -> (queue out=w386:refnum<queue>, error out=w387:errorcluster)  [unwired: 1 in, 1 out]
        n158 = Enqueue Element(queue=w386, element=Install_LV_Events."Exit" ("Install LV Support State"), error in (no error)=w387) -> (error out=w383:errorcluster)  [unwired: 1 in, 2 out]
        n159 = Enqueue Element(queue=w382, element=Install_LV_Events."Exit", error in (no error)=w383) -> (error out=w381:errorcluster)  [unwired: 1 in, 2 out]
      }
      event "Connect": Value Change {
        w393 = T2[] [enum."Connect", enum."Interrogate Device"] items=["Idle", "Connect", "Interrogate Device", "Pre Install", "Add MakerHub Feed", "Update Package Index", "Install LV", "Start LV", "Launch Example", "View Log", "Exit", "Update Hostname", "Menu: Target", "Menu: Install Software", "Menu: Network Settings", "Menu: Target Info", "NIC Select Change", "Menu: Network Settings Save", "Menu: Network Settings Cancel", "Menu: Cancel All"]
        n160 = event-data() -> ()  [unwired: 1 in, 1 out]
        n161 = local write "Connect"(FALSE ("Interrogate")) -> ()
        n162 = for {
          shift-right: [w400] -> w395
          shift-left: w394 -> [w401]
          tunnel: w393 -> [w399] mode=indexing
          tunnel: w392 -> [w398]
          n163 = Enqueue Element(queue=w398, element=w399, error in (no error)=w401) -> (error out=w400:errorcluster)  [unwired: 1 in, 2 out]
        }
      }
      event "Connection": Value Change {
        n164 = event-data() -> ()  [unwired: 1 in, 1 out]
        n165 = Enqueue Element(queue=w402, element=Install_LV_Events."Menu: Target", error in (no error)=w405) -> (error out=w404:errorcluster)  [unwired: 1 in, 2 out]
      }
      event "Installation": Value Change {
        n166 = event-data() -> ()  [unwired: 1 in, 1 out]
        n167 = Enqueue Element(queue=w406, element=Install_LV_Events."Menu: Install Software", error in (no error)=w409) -> (error out=w408:errorcluster)  [unwired: 1 in, 2 out]
      }
      event "Network Settings": Value Change {
        n168 = event-data() -> ()  [unwired: 1 in, 1 out]
        n169 = Enqueue Element(queue=w410, element=Install_LV_Events."Menu: Network Settings", error in (no error)=w413) -> (error out=w412:errorcluster)  [unwired: 1 in, 2 out]
      }
      event "Target Info": Value Change {
        n170 = event-data() -> ()  [unwired: 1 in, 1 out]
        n171 = Enqueue Element(queue=w414, element=Install_LV_Events."Interrogate Device", error in (no error)=w416) -> (error out=w415:errorcluster)  [unwired: 1 in, 2 out]
        n172 = Enqueue Element(queue=w418, element=Install_LV_Events."Menu: Target Info", error in (no error)=w415) -> (error out=w420:errorcluster)  [unwired: 1 in, 2 out]
      }
      event "Network Interface:": Value Change {
        n173 = event-data() -> ()  [unwired: 1 in, 1 out]
        n174 = Enqueue Element(queue=w424, element=Install_LV_Events."NIC Select Change", error in (no error)=w421) -> (error out=w422:errorcluster)  [unwired: 1 in, 2 out]
      }
      event "Network Settings Save": Value Change {
        n175 = event-data() -> ()  [unwired: 1 in, 1 out]
        n176 = Enqueue Element(queue=w427, element=Install_LV_Events."Menu: Network Settings Save", error in (no error)=w428) -> (error out=w425:errorcluster)  [unwired: 1 in, 2 out]
        n177 = local write "Network Settings Save"(FALSE ("Network Settings Save")) -> ()
      }
      event "Network Settings Cancel": Value Change {
        n178 = event-data() -> ()  [unwired: 1 in, 1 out]
        n179 = Enqueue Element(queue=w434, element=Install_LV_Events."Interrogate Device", error in (no error)=w435) -> (error out=w432:errorcluster)  [unwired: 1 in, 2 out]
        n180 = local write "Network Settings Cancel"(FALSE ("Network Settings Save")) -> ()
        n181 = call <vilib>:"Status FGV.vi"("Error In"=w432, "Status"="Cancelling network configuration changes.") -> ("Error Out"=w431:errorcluster)  [unwired: 7 in, 2 out]
      }
      event "Cancel All": Value Change {
        n182 = event-data() -> ()  [unwired: 1 in, 1 out]
        n183 = Enqueue Element(queue=w439, element=Install_LV_Events."Menu: Cancel All", error in (no error)=w440) -> (error out=w437:errorcluster)  [unwired: 1 in, 2 out]
        n184 = local write "Cancel All"(FALSE ("Cancel All")) -> ()
      }
      event "DCHP": Value Change {
        n185 = event-data() -> ("NewVal"=w442:enum32{"DHCP", "Static"})  [unwired: 1 in]
        n186 = case shown="\"DHCP\"" w442 {
          tunnel: w444 -> [w448 w452]
          tunnel: [w447 w451] -> w443
          frame "Static" {
            n187 = call <vilib>:"Set DHCP Status.vi"("Override?"=TRUE, "Error In"=w448, "NIC Mode Override"=NIC_Mode."Static") -> ("Error Out"=w447:errorcluster)  [unwired: 7 in, 1 out]
          }
          frame "DHCP" {
            n188 = call <vilib>:"Set DHCP Status.vi"("Override?"=TRUE, "Error In"=w452, "NIC Mode Override"=NIC_Mode."DHCP") -> ("Error Out"=w451:errorcluster)  [unwired: 7 in, 1 out]
          }
        }
      }
      event "Target Type": Value Change {
        n189 = event-data() -> ("NewVal"=w455:u16)  [unwired: 1 in]
        n190 = case shown="1, Default" w455 {
          tunnel: ["192.168.7.2" ("Hostname or IP:") "raspberrypi" ("Hostname or IP:")] -> w458
          tunnel: ["debian" ("Username:") "pi" ("Username:")] -> w457
          tunnel: ["temppwd" ("Password:") "raspberry" ("Password:")] -> w456
          tunnel: [FALSE TRUE] -> w454
          tunnel: [TRUE FALSE] -> w453
          frame 1, Default {
          }
          frame 0 {
          }
        }
        n191 = local write "Hostname or IP:"(w458) -> ()
        n192 = local write "Username:"(w457) -> ()
        n193 = property on="RPI Info" class="Bool (strict)"("Visible"=w454) -> ()  [unwired: 2 in, 2 out]
        n194 = property on="BBB Info" class="Bool (strict)"("Visible"=w453) -> ()  [unwired: 2 in, 2 out]
        n195 = local write "Password:"(w456) -> ()
      }
      event "Additional installation information:": Value Change {
        n196 = event-data() -> ()  [unwired: 1 in, 4 out]
        n197 = call-poly <vilib>:"Open URL in Default Browser.vi"("error in (no error)"=w470, "URL"="http://www.labviewmakerhub.com" ("Status")) -> ("error out"=w471:errorcluster)  [unwired: 4 in, 1 out]
      }
      event User Event {
        n198 = event-data() -> ()  [unwired: 1 in, 1 out]
      }
    }
  }
  n199 = while {
    tunnel: w10 -> [w483]
    tunnel: w14 -> [w480]
    tunnel: [w478] -> w13
    tunnel: w9 -> [w476]
    tunnel: w6 -> [w475]
    stop <- w481 stop-if-true
    # "Async Events"
    n200 = Dequeue Element(queue=w483, error in (no error)=w480) -> (queue out=w477:refnum<queue>, element=w482:T2, error out=w479:errorcluster)  [unwired: 1 in, 1 out]
    n201 = case shown="\"Idle\", Default" w482 {
      tunnel: [_ _ _ _ _ w501 _ TRUE _] -> w481
      tunnel: w479 -> [w484 w488 w492 w496 w500 w511 w533 w535 w538]
      tunnel: [w484 w486 w490 w494 w498 w506 w532 w535 w537] -> w478
      tunnel: w477 -> [_ _ _ _ _ _ _ _ _]
      tunnel: w476 -> [_ _ _ _ _ w504 _ _ _]
      tunnel: w475 -> [_ _ _ _ _ w505 _ _ _]
      frame "Idle", Default {
      }
      frame "Menu: Target" {
        w485 = enum32{"Target", "Software", "Network"}."Target" ("Tab Control")
        n202 = property on="Tab Control" class="TabCtl (strict)"(error in=w488, "Value"=w485) -> (error out=w487:errorcluster)  [unwired: 1 in, 1 out]
        n203 = call <vilib>:"Update Menu Controls Highlight.vi"("Error In"=w487, "Selected Index"=w485) -> ("Error Out"=w486:errorcluster)  [unwired: 9 in]
      }
      frame "Menu: Install Software" {
        w489 = enum32{"Target", "Software", "Network"}."Software" ("Tab Control")
        n204 = property on="Tab Control" class="TabCtl (strict)"(error in=w492, "Value"=w489) -> (error out=w491:errorcluster)  [unwired: 1 in, 1 out]
        n205 = call <vilib>:"Update Menu Controls Highlight.vi"("Error In"=w491, "Selected Index"=w489) -> ("Error Out"=w490:errorcluster)  [unwired: 9 in]
      }
      frame "Menu: Network Settings" {
        w493 = enum32{"Target", "Software", "Network"}."Network" ("Tab Control")
        n206 = property on="Tab Control" class="TabCtl (strict)"(error in=w496, "Value"=w493) -> (error out=w495:errorcluster)  [unwired: 1 in, 1 out]
        n207 = call <vilib>:"Update Menu Controls Highlight.vi"("Error In"=w495, "Selected Index"=w493) -> ("Error Out"=w494:errorcluster)  [unwired: 9 in]
      }
      frame "Menu: Target Info" {
        w497 = T1."Target Info" ("Tab Control")
        n208 = property on="Tab Control" class="TabCtl (strict)"(error in=w500, "Value"=w497) -> (error out=w499:errorcluster)  [unwired: 1 in, 1 out]
        n209 = call <vilib>:"Update Menu Controls Highlight.vi"("Error In"=w499, "Selected Index"=w497) -> ("Error Out"=w498:errorcluster)  [unwired: 9 in]
      }
      frame "Menu: Cancel All" {
        n210 = Get Queue Status(queue=w504, error in (no error)=w511) -> (queue out=w508:refnum<queue>, error out=w509:errorcluster, # elements in queue=w503:i32)  [unwired: 1 in, 5 out]
        n211 = Greater Than 0?(x=w503) -> (x > 0?=w510:bool)
        n212 = case shown="True" w510 {
          tunnel: w509 -> [w524 w527]
          tunnel: [w524 w527] -> w507
          tunnel: [FALSE ("T button?") w526] -> w502
          frame False {
          }
          frame True {
            n213 = Two Button Dialog(message="Warning: Configuration in process.  Click continue to continue target configuration or quit to abort the configuration process.", 1:"Quit" ("T button name (\"OK\")"), 2:"Continue" ("T button name (\"OK\")")) -> (T button?=w526:bool)
          }
        }
        n214 = case shown="False" w502 {
          tunnel: w508 -> [_ w519]
          tunnel: w507 -> [w512 w518]
          tunnel: [w512 w514] -> w506
          tunnel: w505 -> [_ w521]
          frame True {
          }
          frame False {
            n215 = Flush Queue(queue=w519, error in (no error)=w518) -> (queue out=w516:refnum<queue>, error out=w517:errorcluster)  [unwired: 1 out]
            n216 = Enqueue Element(queue=w516, element=Install_LV_Events."Exit", error in (no error)=w517) -> (error out=w522:errorcluster)  [unwired: 1 in, 2 out]
            n217 = Generate User Event(user event=w521, event data cluster=TRUE ("event data"), error in=w522) -> (error out=w515:errorcluster)  [unwired: 1 in, 1 out]
            n218 = call <vilib>:"Status FGV.vi"("Error In"=w515, "Status"="Aborting current operation...") -> ("Error Out"=w514:errorcluster)  [unwired: 7 in, 2 out]
          }
        }
        n219 = Not(x=w502) -> (.not. x?=w501:bool)
      }
      frame "NIC Select Change" {
        n220 = local read "Network Interface:"() -> (w534:u16)
        n221 = call <vilib>:"Device Data Snapshot FGV.vi"() -> ("Install LV Data"=w531:T3)  [unwired: 4 in]
        n222 = call <vilib>:"Update NIC Ctrls.vi"("Error In"=w533, "Selected NIC"=w534, "Install LV Data"=w531) -> ("Error Out"=w532:errorcluster)  [unwired: 7 in, 1 out]
      }
      frame "Exit" {
      }
      frame "View Log" {
        n223 = Temporary Directory() -> (w546:path)
        n224 = call <vilib>:"Status FGV.vi"("Error In"=w538, "Status FGV State"=Status_FGV_States."Get") -> ("Error Out"=w541:errorcluster, "History"=w539:string)  [unwired: 7 in, 1 out]
        n225 = Build Path(base path=w546, name or relative path="LINX_Log.txt") -> (appended path=w543:path)
        n226 = Path To String(path=w543) -> (string=w545:string)
        n227 = Write to Text File(file (use dialog)=w543, text=w539, error in=w541) -> (error out=w542:errorcluster)  [unwired: 1 in, 2 out]
        n228 = disable-structure shown="TARGET_TYPE==Mac" {
          disable-tunnel: w545 -> [w549 w556 w563]
          disable-tunnel: w542 -> [w548 w555 w562]
          disable-tunnel: [w547 w554 w561] -> w537
          frame condition #0 (active) {
            n229 = Concatenate Strings("cmd /c " ("command line"), w549) -> (w552:string)
            n230 = call <vilib>:"System Exec.vi"("run minimized? (F)"=TRUE, "wait until completion? (T)"=FALSE, "error in (no error)"=w548, "command line"=w552) -> ("error out"=w547:errorcluster)  [unwired: 4 in, 3 out]
          }
          frame condition #1 {
            n231 = Concatenate Strings("open " ("command line"), w556) -> (w559:string)
            n232 = call <vilib>:"System Exec.vi"("run minimized? (F)"=TRUE, "wait until completion? (T)"=FALSE, "error in (no error)"=w555, "command line"=w559) -> ("error out"=w554:errorcluster)  [unwired: 4 in, 3 out]
          }
          frame condition #2 {
            n233 = Concatenate Strings("xdg-open " ("command line"), w563) -> (w566:string)
            n234 = call <vilib>:"System Exec.vi"("run minimized? (F)"=TRUE, "wait until completion? (T)"=FALSE, "error in (no error)"=w562, "command line"=w566) -> ("error out"=w561:errorcluster)  [unwired: 4 in, 3 out]
          }
        }
      }
    }
  }
  n235 = call <vilib>:"SSH Smart Close Session.vi"("Install LV Data"=w17) -> ("Error Out"=w5:errorcluster)  [unwired: 9 in, 1 out]
  n236 = control-ref of="This VI"() -> (w1:refnum<vi>)
  n237 = Merge Errors(w5, w3) -> (w4:errorcluster)
  n238 = call <vilib>:"Close FP.vi"("Error In"=w4, "VI Ref"=w1) -> ("Error Out"=w19:errorcluster)  [unwired: 9 in]
  n239 = Merge Errors(w13, w18, w19) -> (w20:errorcluster)
  n240 = Release Queue(queue=w9, error in (no error)=w20) -> (error out=w12:errorcluster)  [unwired: 1 in, 2 out]
  n241 = Release Queue(queue=w10, error in (no error)=w12) -> (error out=→"Error Out":errorcluster)  [unwired: 1 in, 2 out]
